vi "Write Off-Line.vi"(8 "error in (no error)":errorcluster, 10 "Off-Line":bool, 11 "25-Host Accepts Off-Line in":refnum<class "25-Host Accepts Off-Line.lvclass">) -> (0 "error out":errorcluster, 3 "25-Host Accepts Off-Line out":refnum<class "25-Host Accepts Off-Line.lvclass">)   [LabVIEW 2020, in "SECS Scenarios.lvlib" / "25-Host Accepts Off-Line.lvclass"]
uses:
  25-Host Accepts Off-Line.lvclass
  25-Host Accepts Off-Line.lvclass/25-Host Accepts Off-Line.ctl
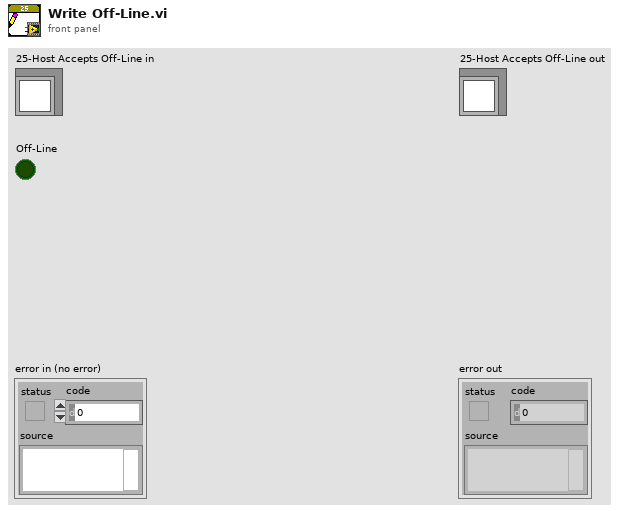
[diagram p1: front panel]
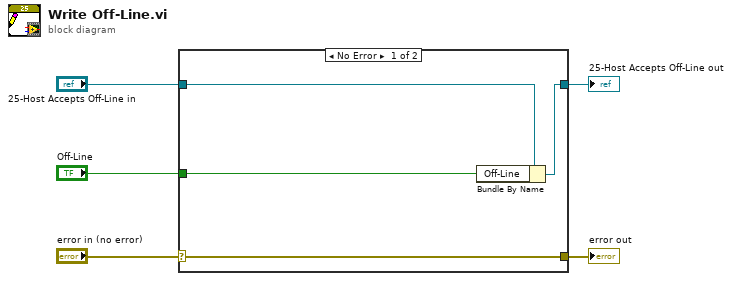
[diagram p0: block diagram]
diagram:
  n1 = case shown="No Error" "error in (no error)" {
    selector: "error in (no error)" -> [w9 w10]
    tunnel: [w9 w10] -> w4
    tunnel: [w7 w11] -> w2
    tunnel: "25-Host Accepts Off-Line in" -> [w8 w11]
    tunnel: "Off-Line" -> [w6 _]
    frame No Error {
      n2 = Bundle By Name(cluster=w8, "Off-Line"=w6) -> (w7:refnum<class "25-Host Accepts Off-Line.lvclass">)
    }
    frame Error {
    }
  }
  "error out" <- w4
  "25-Host Accepts Off-Line out" <- w2
